vi "Load and Apply User Preferences.vi"(8 "error in (no error)":errorcluster) -> (0 "error out":errorcluster, 3 "User Preferences File out":refnum<class "User Preferences File.lvclass">)   [LabVIEW 2020, in "RxnRover.lvlib"]
doc: "Wrapper function to load the user preferences file for Rxn Rover and apply the loaded preferences."
uses:
  RxnRover.lvlib
  User Preferences File.lvclass
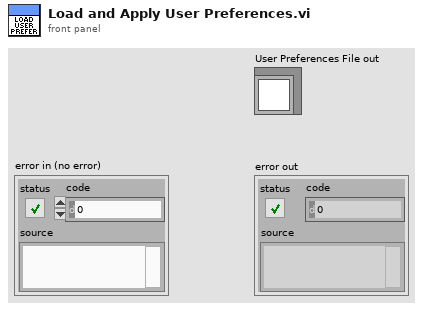
[diagram p1: front panel]
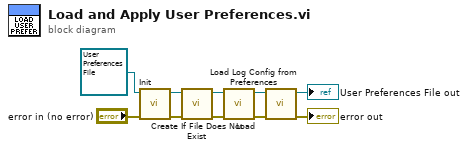
[diagram p0: block diagram]
diagram:
  n1 = call "Init.vi"("error in (no error)"="error in (no error)", "UserPreferencesFileManager in"=refnum<class "User Preferences File.lvclass"> refnum ("User Preferences File.lvclass")) -> ("error out"=w9:errorcluster, "UserPreferencesFileManager out"=w7:refnum<class "User Preferences File.lvclass">)  [unwired: 8 in]
  n2 = call "Create If File Does Not Exist.vi"("error in (no error)"=w9, "User Preferences File in"=w7) -> ("error out"=w10:errorcluster, "User Preferences File out"=w8:refnum<class "User Preferences File.lvclass">)  [unwired: 8 in]
  n3 = call "Load.vi"("error in (no error)"=w10, "User Preferences File in"=w8) -> ("error out"=w4:errorcluster, "User Preferences File out"=w5:refnum<class "User Preferences File.lvclass">)  [unwired: 8 in]
  n4 = call "Load Log Config from Preferences.vi"("error in (no error)"=w4, "User Preferences File in"=w5) -> ("error out"=→"error out":errorcluster, "User Preferences File out"=→"User Preferences File out":refnum<class "User Preferences File.lvclass">)  [unwired: 7 in, 1 out]
